vi "arm autonomous.vi"(0 "Setpoint":dbl) -> (2 "Setpoint Out":dbl, 3 "Done?":bool)   [LabVIEW 2014]
uses:
  global variables/devrefs.vi
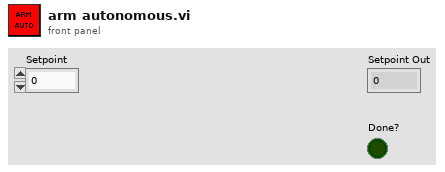
[diagram p1: front panel]
types:
  T1 = typedef "WPI_EncoderDevRef.ctl" = cluster{"DevStatus":errorcluster, "EncoderIndex":T2, "CounterIndex":T3, "DistancePerCount":dbl, "Decoding Type":T4}
  T2 = typedef "FPGA_EncoderIdx.ctl" = enum8{"Enc 0", "Enc 1", "Enc 2", "Enc 3", "Enc 4", "Enc 5", "Enc 6", "Enc 7", "Invalid"}
  T3 = typedef "FPGA_CounterCtrSystemIndex.ctl" = enum8{"Ctr 0", "Ctr 1", "Ctr 2", "Ctr 3", "Ctr 4", "Ctr 5", "Ctr 6", "Ctr 7", "Invalid"}
  T4 = typedef "WPI_EncoderType.ctl" = enum16{"1x", "2x", "4x"}
  T5 = typedef "subStates.ctl" = enum16{"null", "wait", "driver control", "auto", "manual override", "hold position", "rotate", "test", "end"}
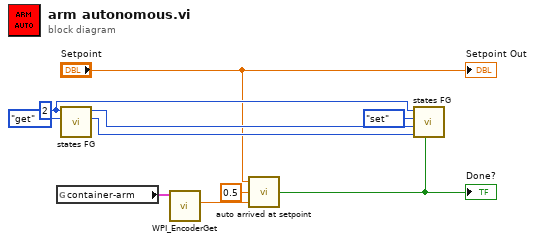
[diagram p0: block diagram]
diagram:
  w9 = 2 ("Loop ID")
  n1 = global read "devrefs.vi" "container-arm"() -> (w3:T1)
  n2 = call "states FG.vi"("menu (get)"=enum16{"set", "get"}."get", "Loop ID"=w9) -> ("state # out"=w7:i32, "subState out"=w8:T5)  [unwired: 6 in, 2 out]
  n3 = call <vilib>:"WPI_EncoderGet.vi"("EncoderDevRef"=w3) -> ("Distance"=w2:dbl)  [unwired: 5 in, 5 out]
  n4 = call "auto arrived at setpoint.vi"("Encoder Distance"=w2, "Tolerance"=0.5, "Setpoint"="Setpoint") -> ("At Location?"=w1:bool)
  "Done?" <- w1
  n5 = call "states FG.vi"("exit in"=w1, "state # in"=w7, "subState in"=w8, "menu (get)"=enum16{"set", "get"}."set", "Loop ID"=w9) -> ()  [unwired: 3 in, 4 out]
  "Setpoint Out" <- "Setpoint"
